vi "PCO_SetAcquireControl.vi"(8 "error in (no error)":errorcluster {"code" format="%x"}, 10 "dwAcquCtrlFlags":u32(ring) items=["ACQUIRE_CONTROL_OFF", "ACQUIRE_CONTROL_FORCE_LOW", "ACQUIRE_CONTROL_FORCE_HIGH"], 11 "ph":u64) -> (0 "error out":errorcluster {"code" format="%x"}, 2 "ErrorMessage":i32 format="%x", 3 "ph out":u64)   [LabVIEW 2019, in "SDK.lvlib" / "RecordingControl.lvlib"]
doc: "<b>Description:</b>\nThis function sets the acquire mode of the camera.\nAcquire mode can be either [auto], [external] or [external modulate].\n\n<b>Supported camera type:</b>\nAll cameras\n\n<b>Descriptor dependency:</b>\ndwGeneralCapsDESC1: NO_ACQUIREMODE"
uses:
  RecordingControl.lvlib
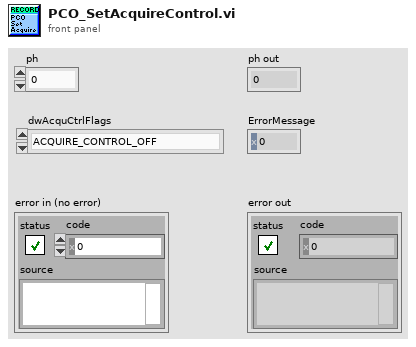
[diagram p1: front panel]
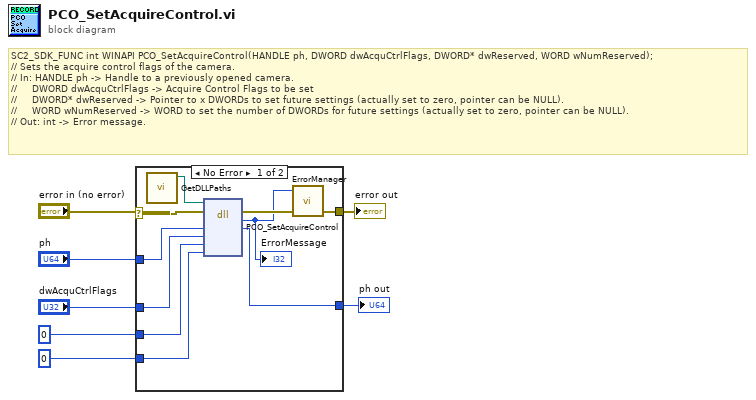
[diagram p0: block diagram]
diagram:
  # "SC2_SDK_FUNC int WINAPI PCO_SetAcquireControl(HANDLE ph, DWORD dwAcquCtrlFlags, DWORD* dwReserved, WORD wNumReserved);\n// Sets the acquire control flags of the camera.\n// In: HANDLE ph -> Handle to a previously opened camera.\n//     DWORD dwAcquCtrlFlags -> Acquire Control Flags to be set\n//     DWORD* dwReserved -> Pointer to x DWORDs to set future settings (actually set to zero, pointer can be NULL).\n//     WORD wNumReserved -> WORD to set the number of DWORDs for future settings (actually set to zero, pointer can be NULL).\n// Out: int -> Error message."
  n1 = case shown="No Error" "error in (no error)" {
    selector: "error in (no error)" -> [w14 w19]
    tunnel: "ph" -> [w17 w18]
    tunnel: [w16 w18] -> w6
    tunnel: "dwAcquCtrlFlags" -> [w15 _]
    tunnel: [w12 w19] -> w4
    tunnel: u32 0 -> [w9 _]
    tunnel: u16 0 -> [w8 _]
    frame No Error {
      n2 = call "GetDLLPaths.vi"() -> ("SC2_Cam_Path"=w10:path)  [unwired: 8 in, 3 out]
      n3 = dll-call lib="?" fn="PCO_SetAcquireControl"(path in=w10, error in=w14, "ph"=w17, "dwAcquCtrlFlags"=w15, "dwReserved"=w9, "wNumReserved"=w8) -> (error out=w13:errorcluster, "return type"=w11:i32, "ph"=w16:u64)  [unwired: 4 in, 1 out]
      "ErrorMessage" <- w11
      n4 = call "ErrorManager.vi"("error in (no error)"=w13, "error code"=w11) -> ("error out"=w12:errorcluster)  [unwired: 2 in, 1 out]
    }
    frame Error {
    }
  }
  "ph out" <- w6
  "error out" <- w4
